vi "VWV Viscosity of Water Vapor (Pa s).vi"(1 "Pure Water Temprature":dbl[unit]) -> (0 "Visocity of  Water Vapor":dbl[unit])   [LabVIEW 2018]
panel:
  out "Visocity of  Water Vapor":dbl[unit](knob) scale=5e-06..1.5e-05
  out "Humidity of Input Air":dbl(knob) scale=0.0..100.0
  in  "RH":dbl
  out "SaiOne":dbl
  out "SaiZero":dbl
  out "Pure Water Temprature":dbl[unit](slide) scale=0.0..100.0
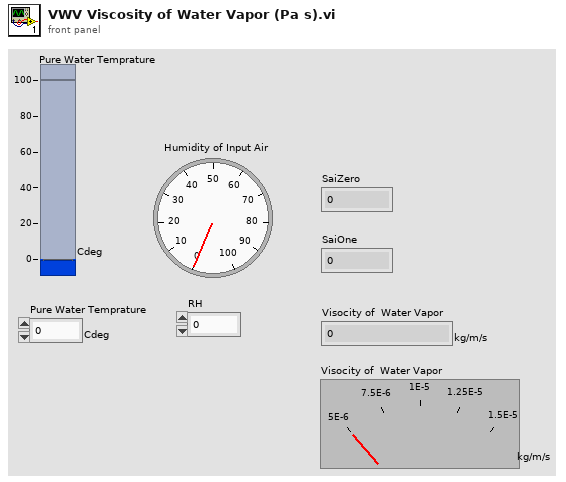
[diagram p1: front panel]
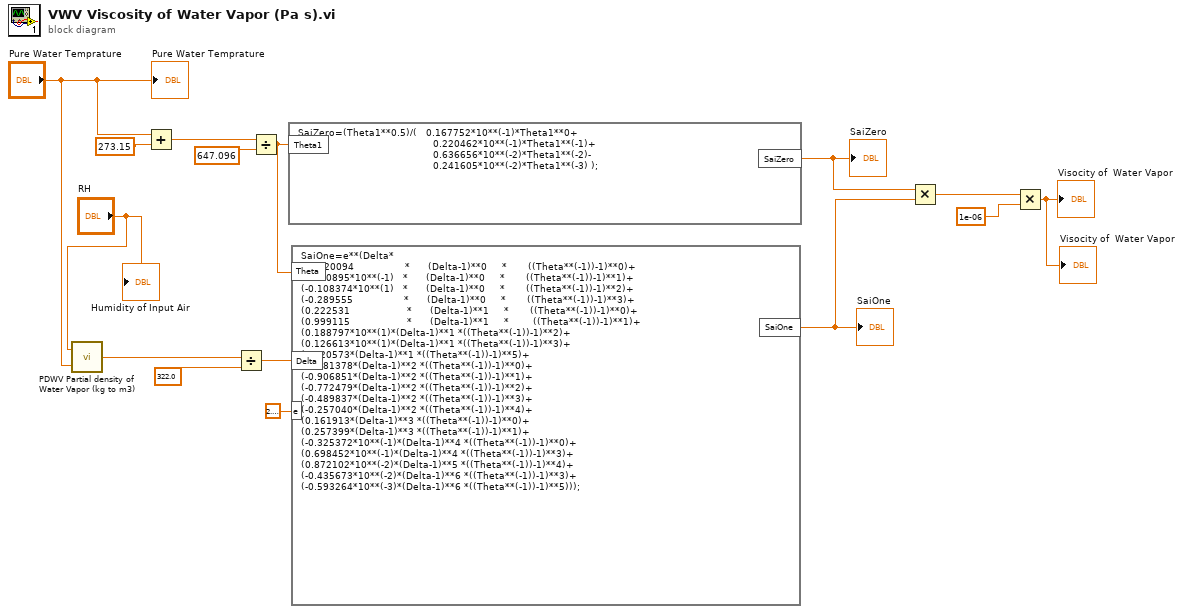
[diagram p0: block diagram]
diagram:
  n1 = call "PDWV Partial density of Water Vapor (kg to m3).vi"("Tceg"="Pure Water Temprature", "RH"="RH") -> ("PDWV"=w10:dbl[unit])
  n2 = Add(x="Pure Water Temprature", y=dbl[unit] 273.15) -> (x+y=w4:dbl[unit])
  n3 = Divide(x=w10, y=dbl[unit] 322.0) -> (x/y=w6:dbl)
  n4 = Divide(x=w4, y=dbl[unit] 647.096) -> (x/y=w3:dbl)
  n5 = formula code="SaiZero=(Theta1**0.5)/(   0.167752*10**(-1)*Theta1**0+\n                                             0.220462*10**(-1)*Theta1**(-1)+\n                                             0.636656*10**(-2)*Theta1**(-2)-\n                                             0.241605*10**(-2)*Theta1**(-3) );"("Theta1"=w3) -> ("SaiZero"=w11:dbl)
  "SaiZero" <- w11
  n6 = formula code="SaiOne=e**(Delta*\n((0.520094                 *      (Delta-1)**0     *       ((Theta**(-1))-1)**0)+\n(0.850895*10**(-1)   *      (Delta-1)**0     *       ((Theta**(-1))-1)**1)+\n(-0.108374*10**(1)   *      (Delta-1)**0     *       ((Theta**(-1))-1)**2)+\n(-0.289555                 *      (Delta-1)**0     *       ((Theta**(-1))-1)**3)+\n(0.222531                   *      (Delta-1)**1     *       ((Theta**(-1))-1)**0)+\n(0.999115                   *      (Delta-1)**1     *        ((Theta**(-1))-1)**1)+\n(0.188797*10**(1)*(Delta-1)**1 *((Theta**(-1))-1)**2)+\n(0.126613*10**(1)*(Delta-1)**1 *((Theta**(-1))-1)**3)+\n(0.120573*(Delta-1)**1 *((Theta**(-1))-1)**5)+\n(-0.281378*(Delta-1)**2 *((Theta**(-1))-1)**0)+\n(-0.906851*(Delta-1)**2 *((Theta**(-1))-1)**1)+\n(-0.772479*(Delta-1)**2 *((Theta**(-1))-1)**2)+\n(-0.489837*(Delta-1)**2 *((Theta**(-1))-1)**3)+\n(-0.257040*(Delta-1)**2 *((Theta**(-1))-1)**4)+\n(0.161913*(Delta-1)**3 *((Theta**(-1))-1)**0)+\n(0.257399*(Delta-1)**3 *((Theta**(-1))-1)**1)+\n(-0.325372*10**(-1)*(Delta-1)**4 *((Theta**(-1))-1)**0)+\n(0.698452*10**(-1)*(Delta-1)**4 *((Theta**(-1))-1)**3)+\n(0.872102*10**(-2)*(Delta-1)**5 *((Theta**(-1))-1)**4)+\n(-0.435673*10**(-2)*(Delta-1)**6 *((Theta**(-1))-1)**3)+\n(-0.593264*10**(-3)*(Delta-1)**6 *((Theta**(-1))-1)**5)));"("Delta"=w6, "e"=2.718281828459045, "Theta"=w3) -> ("SaiOne"=w8:dbl)
  "SaiOne" <- w8
  n7 = Multiply(x=w11, y=w8) -> (x*y=w12:dbl)
  n8 = Multiply(x=w12, y=dbl[unit] 1e-06) -> (x*y=→"Visocity of  Water Vapor" →"Visocity of  Water Vapor":dbl[unit])
  "Pure Water Temprature" <- "Pure Water Temprature"
  "Humidity of Input Air" <- "RH"
